vi "Get Attached Channels.vi"(8 "error in":errorcluster) -> (0 "error out":errorcluster, 2 "Channels":T1[](array[typedef]) {"PCAN Type" items=["Undefined"=0, "PCAN-ISA 82C200"=1, "PCAN-Dongle 82C200"=2, "PCAN-Dongle EPP82C200"=3, "PHYTEC ISA"=4, "PCAN-Dongle SJA1000"=5, "PCAN-Dongle EPP SJA 10000"=6, "PCAN-ISA SJA1000"=9]; "TPCANHandle" items=["PCAN_NONEBUS"=0, "PCAN_USBBUS1"=81, "PCAN_USBBUS2"=82, "PCAN_USBBUS3"=83, "PCAN_USBBUS4"=84, "PCAN_USBBUS5"=85, "PCAN_USBBUS6"=86, "PCAN_USBBUS7"=87, "PCAN_USBBUS8"=88, "PCAN_USBBUS9"=1289, "PCAN_USBBUS10"=1290, "PCAN_USBBUS11"=1291, "PCAN_USBBUS12"=1292, "PCAN_USBBUS13"=1293, "PCAN_USBBUS14"=1294, "PCAN_USBBUS15"=1295, "PCAN_USBBUS16"=1296]}, 5 "TPCANStatus":T4 items=["PCAN_ERROR_OK"=0, "PCAN_ERROR_XMTFULL"=1, "PCAN_ERROR_OVERRUN"=2, "PCAN_ERROR_BUSLIGHT"=4, "PCAN_ERROR_BUSHEAVY"=8, "PCAN_ERROR_BUSPASSIVE"=262144, "PCAN_ERROR_BUSOFF"=16, "PCAN_ERROR_QRCVEMPTY"=32, "PCAN_ERROR_QOVERRUN"=64, "PCAN_ERROR_QXMTFULL"=128, "PCAN_ERROR_REGTEST"=256, "PCAN_ERROR_NODRIVER"=512, "PCAN_ERROR_HWINUSE"=1024, "PCAN_ERROR_NETINUSE"=2048, "PCAN_ERROR_ILLHW"=5120, "PCAN_ERROR_ILLNET"=6144, "PCAN_ERROR_ILLCLIENT"=7168, "PCAN_ERROR_RESOURCE"=8192, "PCAN_ERROR_ILLPARAMTYPE"=16384, "PCAN_ERROR_ILLPARAMVAL"=32768, "PCAN_ERROR_UNKNOWN"=65536, "PCAN_ERROR_ILLDATA"=131072, "PCAN_ERROR_ILLMODE"=524288, "PCAN_ERROR_CAUTION"=33554432, "PCAN_ERROR_INITIALIZE"=67108864, "PCAN_ERROR_ILLOPERATION"=134217728])   [LabVIEW 2018, in "PCANBasic.lvlib"]
doc: "This parameter is used to get information about all existing PCAN channels on a system in a single call, regardless of their current availability (See CHANNEL_CONDITION)."
uses:
  PCANBasic.lvlib
  TPCANParameter.ctl
  TPCANHandle.ctl
  TPCANChannelInformation.ctl
  PCAN Type.ctl
  TPCANStatus.ctl
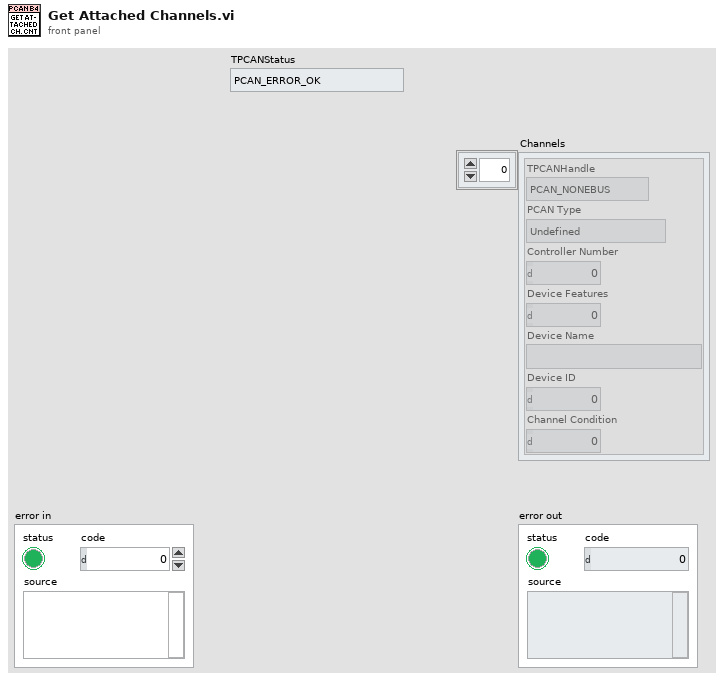
[diagram p1: front panel]
types:
  T1 = typedef "PCANBasic.lvlib/TPCANChannelInformation.ctl" = cluster{"TPCANHandle":T2, "PCAN Type":T3, "Controller Number":u8, "Device Features":u32, "Device Name":string, "Device ID":u32, "Channel Condition":u32}
  T2 = typedef "PCANBasic.lvlib/TPCANHandle.ctl" = u16
  T3 = typedef "PCANBasic.lvlib/PCAN Type.ctl" = u8
  T4 = typedef "PCANBasic.lvlib/TPCANStatus.ctl" = u32
  T5 = typedef "PCANBasic.lvlib/TPCANParameter.ctl" = enum16{"Unknown", "PCAN_DEVICE_ID", "PCAN_5VOLTS_POWER", "PCAN_RECEIVE_EVENT", "PCAN_MESSAGE_FILTER", "PCAN_API_VERSION", "PCAN_CHANNEL_VERSION", "PCAN_BUSOFF_AUTORESET", "PCAN_LISTEN_ONLY", "PCAN_LOG_LOCATION", "PCAN_LOG_STATUS", "PCAN_LOG_CONFIGURE", "PCAN_LOG_TEXT", "PCAN_CHANNEL_CONDITION", "PCAN_HARDWARE_NAME", "PCAN_RECEIVE_STATUS", "PCAN_CONTROLLER_NUMBER", "PCAN_TRACE_LOCATION", "PCAN_TRACE_STATUS", "PCAN_TRACE_SIZE", "PCAN_TRACE_CONFIGURE", "PCAN_CHANNEL_IDENTIFYING", "PCAN_CHANNEL_FEATURES", "PCAN_BITRATE_ADAPTING", "PCAN_BITRATE_INFO", "PCAN_BITRATE_INFO_FD", "PCAN_BUSSPEED_NOMINAL", "PCAN_BUSSPEED_DATA", "PCAN_IP_ADDRESS", "PCAN_LAN_SERVICE_STATUS", "PCAN_ALLOW_STATUS_FRAMES", "PCAN_ALLOW_RTR_FRAMES", "PCAN_ALLOW_ERROR_FRAMES", "PCAN_INTERFRAME_DELAY", "PCAN_ACCEPTANCE_FILTER_11BIT", "PCAN_ACCEPTANCE_FILTER_29BIT", "PCAN_IO_DIGITAL_CONFIGURATION", "PCAN_IO_DIGITAL_VALUE", "PCAN_IO_DIGITAL_SET", "PCAN_IO_DIGITAL_CLEAR", "PCAN_IO_ANALOG_VALUE", "PCAN_FIRMWARE_VERSION", "PCAN_ATTACHED_CHANNELS_COUNT", "PCAN_ATTACHED_CHANNELS", "PCAN_ALLOW_ECHO_FRAMES", "PCAN_DEVICE_PART_NUMBER", "PCAN_HARD_RESET_STATUS", "PCAN_LAN_CHANNEL_DIRECTION", "PCAN_DEVICE_GUID"}
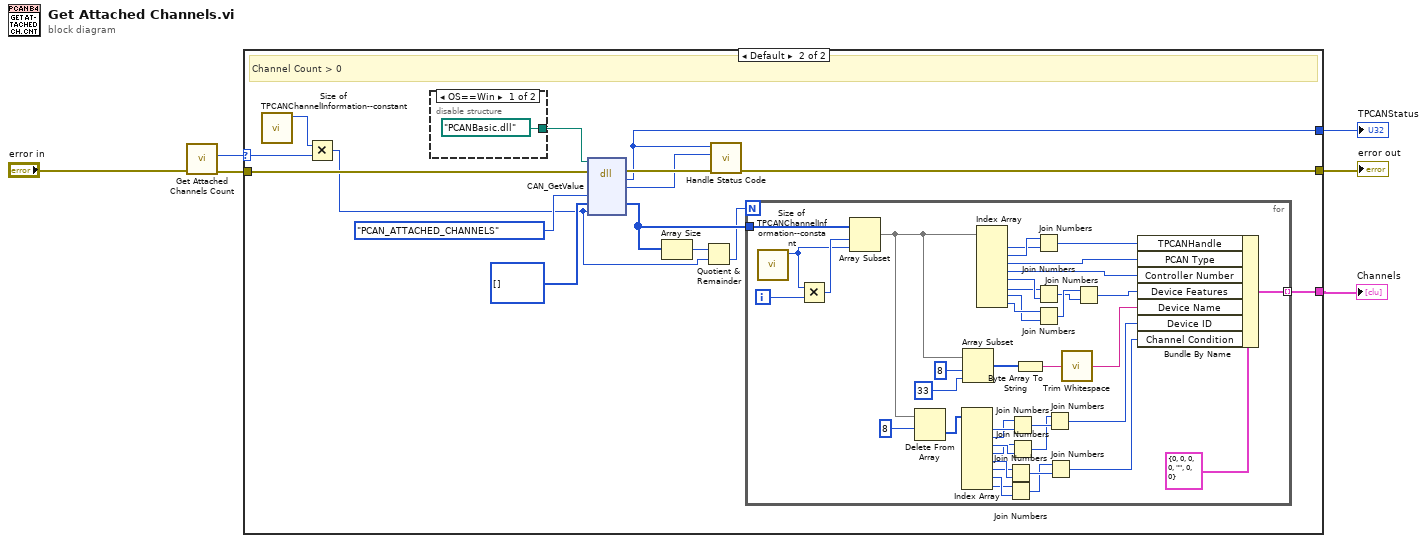
[diagram p0: block diagram]
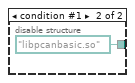
[diagram p3: hidden frame]
diagram:
  n1 = call "Get Attached Channels Count.vi"("error in"="error in") -> ("error out"=w3:errorcluster, "Channels Count"=w2:u32)  [unwired: 8 in, 1 out]
  n2 = case shown="Default" w2 {
    selector: w2 -> [_ w14]
    tunnel: [w7 w19] -> w6
    tunnel: [_ w18] -> w5
    tunnel: w3 -> [w7 w16]
    tunnel: [_ w8] -> w1
    frame 0 {
      # "Channel Count = 0"
    }
    frame Default {
      # "Channel Count > 0"
      n3 = call "Size of TPCANChannelInformation--constant.vi"() -> ("Size of TPCANChannelInformation"=w15:u32)  [unwired: 11 in]
      n4 = Multiply(x=w15, y=w14) -> (x*y=w11:u32)
      n5 = disable-structure shown="OS==Win" {
        disable-tunnel: [path "PCANBasic.dll" path "libpcanbasic.so"] -> w22
        frame condition #0 (active) {
        }
        frame condition #1 {
        }
      }
      n6 = dll-call lib="?" fn="CAN_GetValue"(path in=w22, error in=w16, "TPCANParameter"=TPCANParameter."PCAN_ATTACHED_CHANNELS", "Buffer"=u8[] [], "BufferLength"=w11) -> (error out=w21:errorcluster, "TPCANStatus"=w18:u32, "Channel"=w17:u16, "Buffer"=w10:u8[])  [unwired: 4 in, 1 out]
      n7 = Array Size(array=w10) -> (size(s)=w12:i32)
      n8 = Quotient & Remainder(x=w12, y=w11) -> (floor(x/y)=w9:u32)  [unwired: 1 out]
      n9 = call "Handle Status Code.vi"("error in"=w21, "TPCANHandle"=w17, "TPCANStatus"=w18) -> ("error out"=w19:errorcluster)  [unwired: 8 in]
      n10 = for {
        N: w9 -> [_]
        tunnel: w10 -> [w62]
        tunnel: [w26] -> w8 mode=indexing
        i -> [w61]
        n11 = call "Size of TPCANChannelInformation--constant.vi"() -> ("Size of TPCANChannelInformation"=w59:u32)  [unwired: 11 in]
        n12 = Multiply(x=w59, y=w61) -> (x*y=w60:u32)
        n13 = Array Subset(array=w62, index=w60, length=w59) -> (w24:u8[])
        n14 = Delete From Array(array=w24, length=8) -> (deleted portion=w23:u8[])  [unwired: 1 in, 1 out]
        n15 = Index Array(array=w23) -> (element #1=w38:u8, element #2=w37:u8, element #3=w40:u8, element #4=w39:u8, element #5=w42:u8, element #6=w41:u8, element #7=w44:u8, element #8=w43:u8)  [unwired: 8 in]
        n16 = Array Subset(array=w24, index=8, length=33) -> (w28:u8[])
        n17 = Index Array(array=w24) -> (element #1=w56:u8, element #2=w57:u8, element #3=w54:u8, element #4=w53:u8, element #5=w52:u8, element #6=w51:u8, element #7=w46:u8, element #8=w47:u8)  [unwired: 8 in]
        n18 = Join Numbers(hi=w41, lo=w42) -> ((hi.lo)=w36:u16)
        n19 = Join Numbers(hi=w43, lo=w44) -> ((hi.lo)=w35:u16)
        n20 = Join Numbers(hi=w37, lo=w38) -> ((hi.lo)=w34:u16)
        n21 = Join Numbers(hi=w39, lo=w40) -> ((hi.lo)=w33:u16)
        n22 = Byte Array To String(unsigned byte array=w28) -> (string=w27:string)
        n23 = Join Numbers(hi=w57, lo=w56) -> ((hi.lo)=w55:u16)
        n24 = Join Numbers(hi=w51, lo=w52) -> ((hi.lo)=w49:u16)
        n25 = Join Numbers(hi=w47, lo=w46) -> ((hi.lo)=w50:u16)
        n26 = Join Numbers(hi=w33, lo=w34) -> ((hi.lo)=w32:u32)
        n27 = Join Numbers(hi=w35, lo=w36) -> ((hi.lo)=w31:u32)
        n28 = call <vilib>:"Trim Whitespace.vi"("string"=w27) -> ("trimmed string"=w25:string)  [unwired: 1 in]
        n29 = Join Numbers(hi=w50, lo=w49) -> ((hi.lo)=w48:u32)
        n30 = Bundle By Name(cluster=T1 {"TPCANHandle"=0, "PCAN Type"=0, "Controller Number"=0, "Device Features"=0, "Device Name"="", "Device ID"=0, "Channel Condition"=0} ("TPCANChannelInformation"), "TPCANHandle"=w55, "PCAN Type"=w54, "Controller Number"=w53, "Device Features"=w48, "Device Name"=w25, "Device ID"=w32, "Channel Condition"=w31) -> (w26:T1)
      }
    }
  }
  "error out" <- w6
  "TPCANStatus" <- w5
  "Channels" <- w1
